vi "Robot Global Data.vi"() -> ()   [LabVIEW 2016]
doc: "This global VI can contain as many global variables as you need. Place a control on the panel, give it a good name. To read or write to it from a VI, drag the icon to the diagram of that VI. You can also drag from the project. Click on the node to change which global you access. You shouldn't have multiple locations writing to a global or it will cause a race-condition."
uses:
  <vilib>/Rock Robotics/WPI/Camera/WPI_CameraImageSize.ctl
  <vilib>/Rock Robotics/WPI/DriverStation/WPI_DriverStationRobotMode2.ctl
  Common Code/Intake Command Cluster.ctl
  Common Code/Intake Mode.ctl
  Common Code/Intake Commands.ctl
  Common Code/Dashboard Packet.ctl
  Common Code/Intake Presets.ctl
panel:
  in  "Dashboard Packet":T1
  in  "Intake Command Cluster":T3
  in  "Robot Mode":T6
  in  "image size":T7=enum."320x240"
  in  "Enable Vision":bool
  # "Intake"
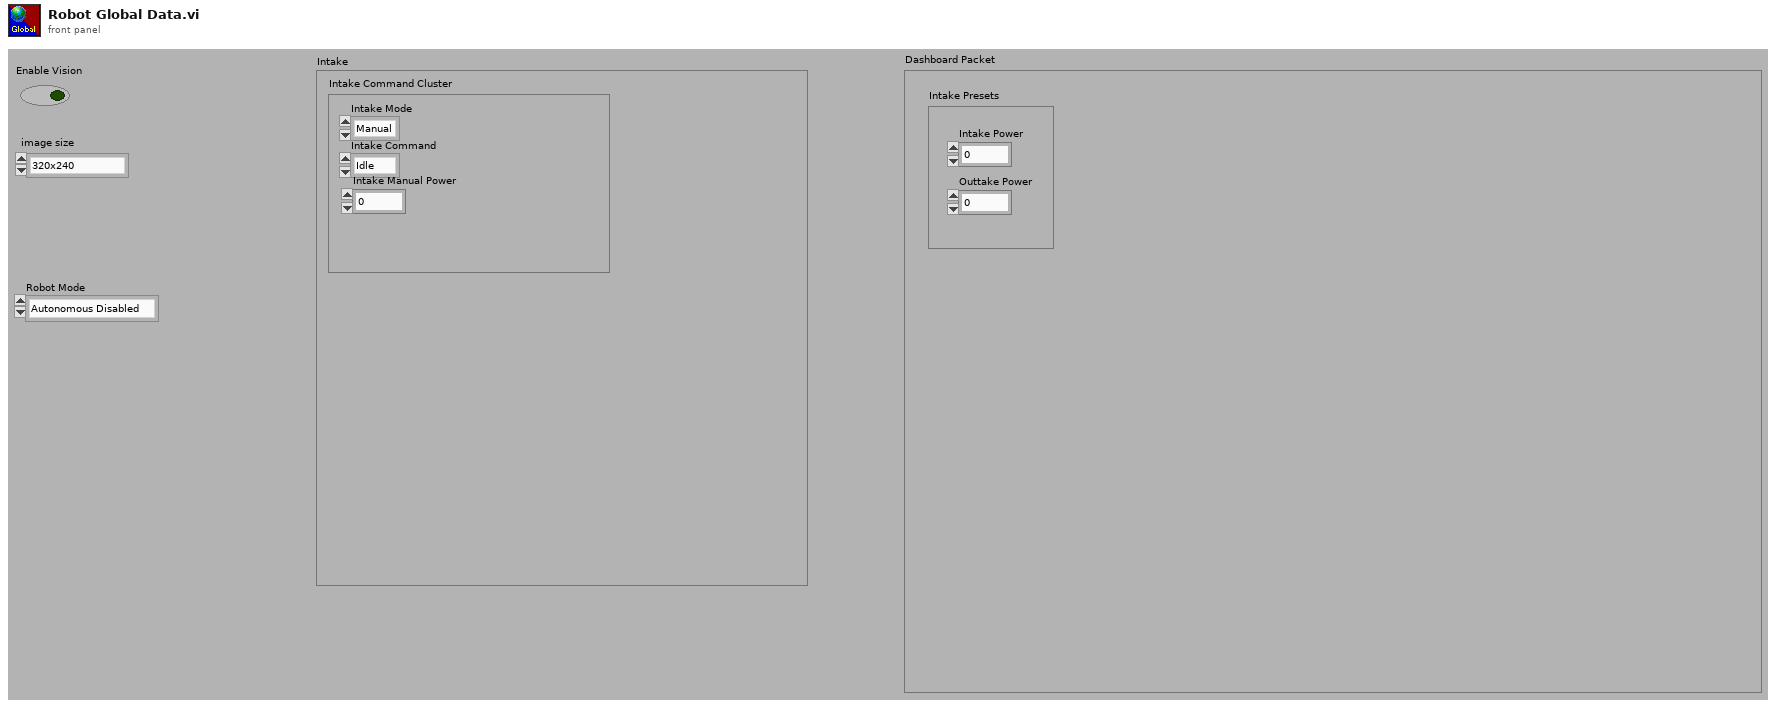
[diagram p1: front panel]
types:
  T1 = typedef "Dashboard Packet.ctl" = cluster{"Intake Presets":T2}
  T2 = typedef "Intake Presets.ctl" = cluster{"Intake Power":dbl, "Outtake Power":dbl}
  T3 = typedef "Intake Command Cluster.ctl" = cluster{"Intake Mode":T4, "Intake Command":T5, "Intake Manual Power":dbl}
  T4 = typedef "Intake Mode.ctl" = enum16{"Manual", "Auto"}
  T5 = typedef "Intake Commands.ctl" = enum16{"Idle", "Intake", "Outtake"}
  T6 = typedef "WPI_DriverStationRobotMode2.ctl" = enum16{"Autonomous Disabled", "Autonomous Enabled", "Teleop Disabled", "Teleop Enabled", "Disconnected", "Finish", "Test Disabled", "Test Enabled", "Emergency Stopped"}
  T7 = typedef "WPI_CameraImageSize.ctl" = enum16{"640x480", "320x240", "160x120", "Custom"}
diagram:
